vi "GetSerializableData.vi"(8 "error in (no error)":errorcluster, 9 "Options":T1, 10 "Data in":T3, 11 "DNL_LabVIEW Object in":refnum<class "BlueSerializableTemplate.lvclass">) -> (0 "error out":errorcluster, 2 "Data out":T3, 3 "DNL_LabVIEW Object out":refnum<class "BlueSerializableTemplate.lvclass">)   [LabVIEW 2020, in "BlueSerializableTemplate.lvlib" / "BlueSerializableTemplate.lvclass"]
doc: "Dynamic Dispatch VI which returns a variant of an entire inheritance heirarchy's serializable data which can later be serialized by a <b>SerializerBase</b> into any format."
uses:
  BlueSerializableTemplate.lvclass
  BlueSerializer/Support/GetSerializableDataCluster.ctl
  BlueSerializer/GetSerializableDataAction.ctl
  BlueSerializer/Support/GetSerializableDataClusterClass.ctl
  BlueSerializer/Support/SerializableDataGetDataAction.ctl
  BlueSerializer/ClassNameAndVersion.ctl
  <vilib>/Utility/EditLVLibs/LibVersion.ctl
  BlueSerializer/SerializeOptionsPayload.ctl
  BlueSerializer/SerializeOptions.ctl
  BlueSerializer/ClassNameCacheMap.ctl
  BlueSerializer/ClassNameObj.ctl
  BlueSerializableTemplate.lvclass/BlueSerializableTemplate.ctl
  BlueSerializer/CheckIfPlaceholder.vi
  <vilib>/Utility/Data Type/Get Type Information.vi
  <vilib>/Utility/Data Type/Get Cluster Information.vi
  BlueSerializer/Support/Anything_To_Variant.vi
  <userlib>/_OpenG.lib/lvdata/lvdata.llb/Set Data Name__ogtk.vi
  BlueSerializable/BlueSerializable.lvclass
  BlueSerializer/BlueSerializer.lvclass
  <vilib>/Utility/EditLVLibs/Edit LVLibs.lvlib
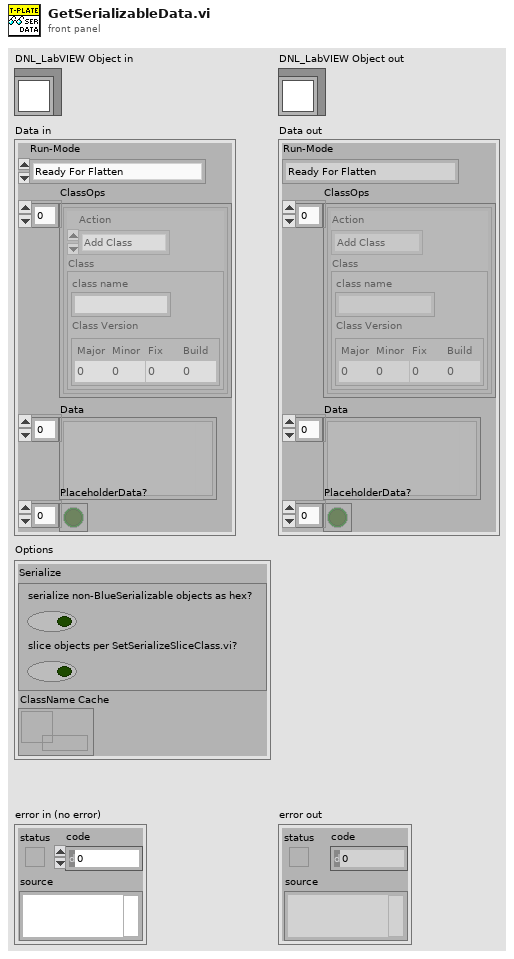
[diagram p1: front panel]
types:
  T1 = typedef "BlueSerialization.lvlib/BlueSerializer.lvclass/SerializeOptionsPayload.ctl" = cluster{"Serialize":T2, "ClassName Cache":refnum<data-value>}
  T2 = typedef "BlueSerialization.lvlib/BlueSerializer.lvclass/SerializeOptions.ctl" = cluster{"serialize non-BlueSerializable objects as hex?":bool, "slice objects per SetSerializeSliceClass.vi?":bool}
  T3 = typedef "BlueSerialization.lvlib/BlueSerializer.lvclass/GetSerializableDataCluster.ctl" = cluster{"Run-Mode":T4, "ClassOps":T5[], "Data":variant[], "PlaceholderData?":bool[]}
  T4 = typedef "BlueSerialization.lvlib/BlueSerializer.lvclass/GetSerializableDataAction.ctl" = enum16{"Ready For Flatten", "Unmodified Data Access"}
  T5 = typedef "BlueSerialization.lvlib/BlueSerializer.lvclass/GetSerializableDataClusterClass.ctl" = cluster{"Action":T6, "Class":T7}
  T6 = typedef "BlueSerialization.lvlib/BlueSerializer.lvclass/SerializableDataGetDataAction.ctl" = enum16{"Add Class", "Drop Class"}
  T7 = typedef "BlueSerialization.lvlib/BlueSerializer.lvclass/ClassNameAndVersion.ctl" = cluster{"class name":string, "Class Version":T8}
  T8 = typedef "Edit LVLibs.lvlib/LibVersion.ctl" = cluster{"Major":u16, "Minor":u16, "Fix":u16, "Build":u16}
  T9 = typedef "BlueSerializableTemplate.lvlib/BlueSerializableTemplate.lvclass/SerializableData.ctl" = cluster{"Placeholder":bool}
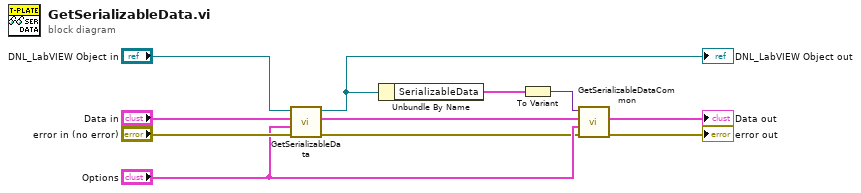
[diagram p0: block diagram]
diagram:
  n1 = call-parent "GetSerializableData.vi"("error in (no error)"="error in (no error)", "Options"="Options", "Data in"="Data in", "BlueSerializable in"="DNL_LabVIEW Object in") -> ("error out"=w3:errorcluster, "Data out"=w2:T3, "BlueSerializable out"=w8:refnum<class "BlueSerializableTemplate.lvclass">)  [unwired: 5 in]
  "DNL_LabVIEW Object out" <- w8
  n2 = Unbundle By Name(w8) -> ("SerializableData"=w4:T9)
  n3 = To Variant(anything=w4) -> (Variant=w1:variant)
  n4 = call "GetSerializableDataCommon.vi"("error in (no error)"=w3, "Options"="Options", "Data (FromParent)"=w2, "SerializableData"=w1) -> ("error out"=→"error out":errorcluster, "Data"=→"Data out":T3)  [unwired: 6 in]
